vi "Get Waveform AI Channel.vi"(8 "error in (no error)":errorcluster, 11 "Reference in":waveform(dbl)) -> (0 "error out":errorcluster, 2 "AI Channel":i32, 3 "Reference out":waveform(dbl))   [LabVIEW 2019, in "Instrument.DAQ.lvclass"]
uses:
  Instrument.DAQ.lvclass
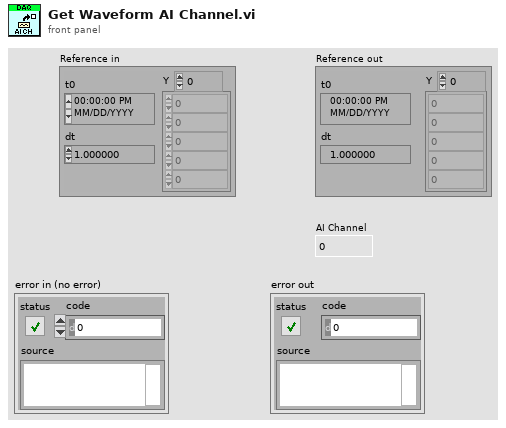
[diagram p1: front panel]
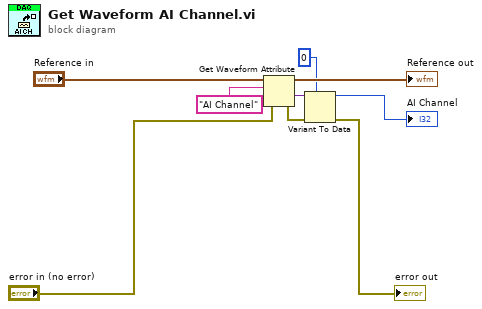
[diagram p0: block diagram]
diagram:
  n1 = Get Waveform Attribute(4:"error in (no error)", 6:"AI Channel" ("name"), 7:"Reference in") -> (0:w1:errorcluster, 1:w2:variant, 3:→"Reference out":waveform(dbl))  [unwired: 1 in, 1 out]
  n2 = Variant To Data(error in=w1, type=0 ("Reference"), Variant=w2) -> (data=→"AI Channel":i32, error out=→"error out":errorcluster)
